vi "Index Array (String Value).vi"(8 "error in (no error)":errorcluster, 9 "index":i32, 10 "JSON Array in":refnum<class "JSON Array.lvclass">) -> (0 "error out":errorcluster, 1 "String":string)   [LabVIEW 2015, in "LVJSON.lvlib" / "JSON Array.lvclass"]
doc: "Returns the String value of the JSON String element of the JSON array at index."
uses:
  JSON Array.lvclass
  JSON String/Read value (String).vi
  Index Array (String).vi
  JSON Basic Type/JSON Literal.lvclass
  JSON String/JSON String.lvclass
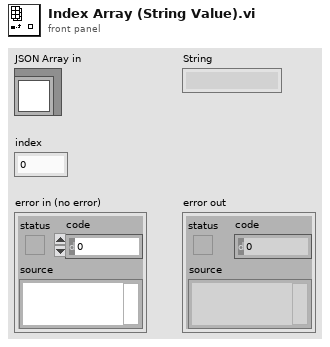
[diagram p1: front panel]
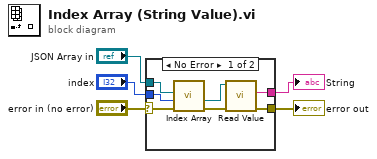
[diagram p0: block diagram]
diagram:
  n1 = case shown="No Error" "error in (no error)" {
    selector: "error in (no error)" -> [w8 w13]
    tunnel: [w9 w13] -> w4
    tunnel: "JSON Array in" -> [w7 _]
    tunnel: "index" -> [w6 _]
    tunnel: [w10 _] -> w1
    frame No Error {
      n2 = call-poly "Index Array.vi"("error in (no error)"=w8, "index"=w6, "JSON Array in"=w7) -> ("error out"=w11:errorcluster, "JSON String"=w12:refnum<class "JSON String.lvclass">)  [unwired: 7 in]
      n3 = call-poly "Read Value.vi"("error in (no error)"=w11, "JSON String in"=w12) -> ("error out"=w9:errorcluster, "value"=w10:string)  [unwired: 8 in]
    }
    frame Error {
    }
  }
  "error out" <- w4
  "String" <- w1
